vi "Marker Line Width Write.vi"(4 "error in (no error)":errorcluster, 5 "Value":u8, 6 "Container State":T3, 7 "Display State In":T1) -> (0 "error out":errorcluster, 3 "Display State Out":T1)   [LabVIEW 2017, in "2D Error Bar.xctl"]
uses:
  <vilib>/Math Plots/2D Math Plots/2D Error Bar/2D Error Bar XCtrl/2D Error Bar.xctl
  <vilib>/_xctls/Container State.ctl
  <vilib>/Math Plots/2D Math Plots/2D Error Bar/2D Error Bar XCtrl/State.ctl
  <vilib>/Math Plots/2D Math Plots/2D Error Bar/2D Error Bar/2D Error Bar.lvclass
  e:/builds/penguin/labview/branches/2017/dev/dist/vi.lib/Math Plots/2D Math Plots/2D Plot/2D Plot/2D Plot.lvclass
  <vilib>/Math Plots/2D Math Plots/2D Plot/Action String/2DMathPlot Ctrl Act Queue.ctl
  <vilib>/Math Plots/2D Math Plots/2D Plot/Action String/2DMathPlot Ctrl Act Cluster.ctl
  <vilib>/Math Plots/2D Math Plots/2D Plot/Action String/2DMathPlot State Class.ctl
  <vilib>/Math Plots/2D Math Plots/2D Plot/2D Plot/2D Plot.lvclass
  <vilib>/_xctls/XControlSupport.lvlib
panel:
  # "Replace the Value Control below with a Control of desired type.\nDo not remove this Control or the others from the connector pane.\nDo not change the connector pane pattern.\nThe Value control should always be the third terminal from top on the input side in the connector pane."
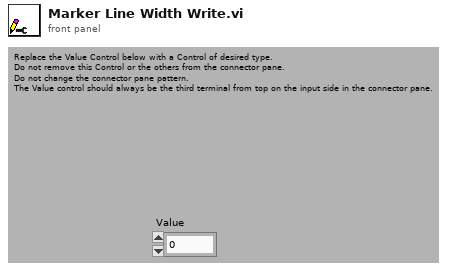
[diagram p1: front panel]
types:
  T1 = typedef "2D Error Bar.xctl/State.ctl" = cluster{"2D Error Bar.lvclass":refnum<class "2D Error Bar.lvclass">, "Control Ref Queue":T2, "Main Frame Color":u32, "Plot Legend Color":u32}
  T2 = typedef "2DMathPlot Ctrl Act Queue.ctl" = refnum<queue>
  T3 = typedef "XControlSupport.lvlib/Container State.ctl" = cluster{"Indicator?":bool, "Run Mode?":bool, " Refnum":refnum<vi>}
  T4 = typedef "2DMathPlot State Class.ctl" = enum16{"Update All (Undo)", "Update General", "Update Appearance", "Update Format", "Update Scale", "Update Marker", "Update Cursor", "None"}
  T5 = typedef "2D Error Bar.lvclass/2D Error Bar Property Array.ctl" = T6[]
  T6 = typedef "2D Error Bar.lvclass/2D Error Bar Property.ctl" = cluster{"Marker Size":dbl, "Marker Line Style":u8, "Marker Line Width":u8, "Marker Color":u32, "Error Bar Interpolation":enum16{"Show Point", "Show Line", "Show Bar"}, "Error Mode":enum16{"Show Y Error", "Show X Error", "Show Both Error"}}
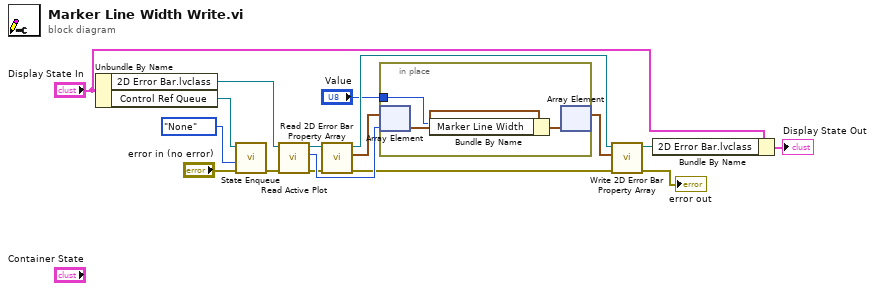
[diagram p0: block diagram]
diagram:
  n1 = Unbundle By Name("Display State In") -> ("2D Error Bar.lvclass"=w17:refnum<class "2D Error Bar.lvclass">, "Control Ref Queue"=w7:T2)
  n2 = call <vilib>:"State Enqueue.vi"("error in (no error)"="error in (no error)", "Display State Change Class"=2DMathPlot_State_Class."None", "Control Ref Queue"=w7) -> ("error out"=w6:errorcluster)  [unwired: 8 out]
  n3 = call <vilib>:"Read Active Plot.vi"("error in (no error)"=w6, "2D Plot.lvclass in"=w17) -> ("error out"=w12:errorcluster, "Active Plot"=w13:i32, "2D Plot.lvclass out"=w16:refnum<class "2D Error Bar.lvclass">)  [unwired: 7 out]
  n4 = call <vilib>:"Read 2D Error Bar Property Array.vi"("error in (no error)"=w12, "2D Error Bar.lvclass in"=w16) -> ("error out"=w10:errorcluster, "2D Error Bar Property Array"=w11:T5, "2D Error Bar.lvclass out"=w15:refnum<class "2D Error Bar.lvclass">)  [unwired: 7 out]
  n5 = in-place {
    in-place-border: "Value" -> [w18]
    n6 = in-place-array #1(w11, w13) -> (w20:T6)
    n7 = Bundle By Name(cluster=w20, "Marker Line Width"=w18) -> (w19:T6)
    n8 = in-place-array #1(w19) -> (w9:T5)  [unwired: 1 out]
  }
  n9 = call <vilib>:"Write 2D Error Bar Property Array.vi"("error in (no error)"=w10, "2D Error Bar Property Array"=w9, "2D Error Bar.lvclass in"=w15) -> ("error out"=→"error out":errorcluster, "2D Error Bar.lvclass out"=w14:refnum<class "2D Error Bar.lvclass">)  [unwired: 1 in, 6 out]
  n10 = Bundle By Name(cluster="Display State In", "2D Error Bar.lvclass"=w14) -> (→"Display State Out":T1)
